vi "NI9234_SUB-VI_UserEvent.vi"(6 "Method_UsE":T3, 8 "error in (no error)":errorcluster, 11 "Cluster_UserEvent":T1) -> (0 "error out":errorcluster, 3 "user event out":refnum<user-event>)   [LabVIEW 2020]
uses:
  TYPEDEF/NI9234_TD_MethodSendEventEvent.ctl
  TYPEDEF/NI9234_TD_ClusterGUIEvents.ctl
  TYPEDEF/NI9234_TD_MethodEvent.ctl
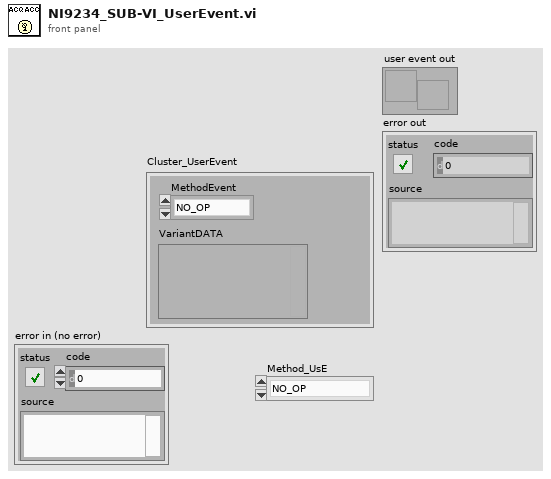
[diagram p1: front panel]
types:
  T1 = typedef "NI9234_TD_ClusterGUIEvents.ctl" = cluster{"MethodEvent":T2, "VariantDATA":variant}
  T2 = typedef "NI9234_TD_MethodEvent.ctl" = enum16{"NO_OP", "EVENTO", "ZERO_POS_REL", "ENABLE_CICLI", "CICLI_ESTENSIONE", "CICLI_RETROAZIONE", "CICLI_Numero", "CICLI_GoToMin", "CICLI_ABORT"}
  T3 = typedef "NI9234_TD_MethodSendEventEvent.ctl" = enum16{"NO_OP", "INIT", "SEND", "CLOSE"}
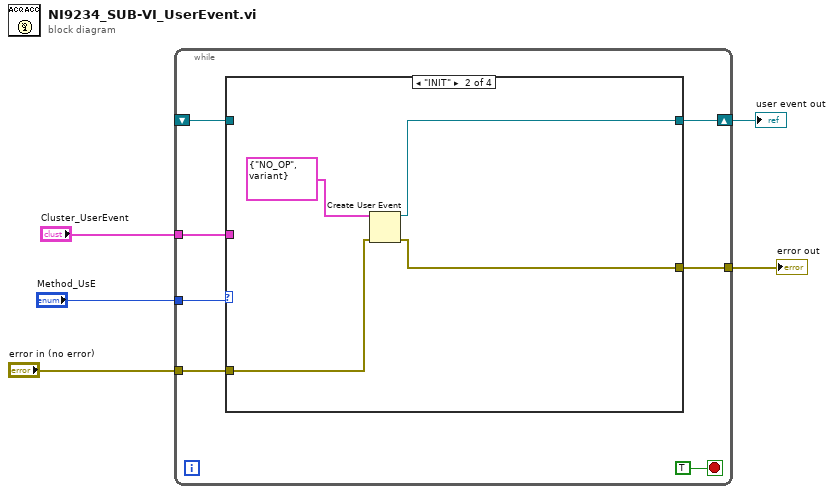
[diagram p0: block diagram]
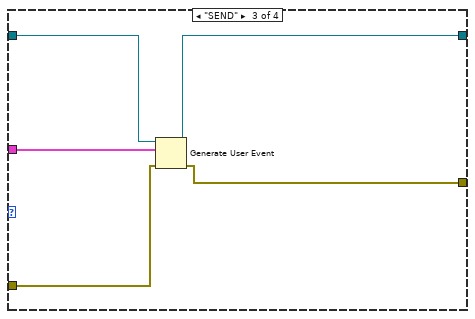
[diagram p3: hidden frame]
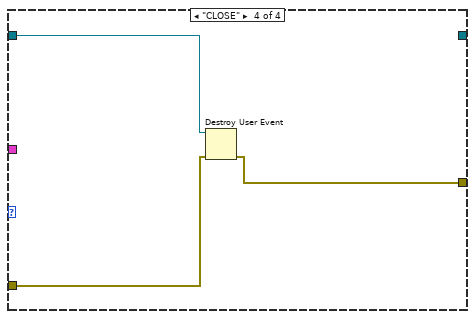
[diagram p4: hidden frame]
diagram:
  n1 = while {
    tunnel: "Method_UsE" -> [w11]
    tunnel: "Cluster_UserEvent" -> [w10]
    shift-right: [w9] -> w3
    shift-left: _ -> [w8]
    tunnel: [w7] -> w2
    tunnel: "error in (no error)" -> [w6]
    stop <- TRUE stop-if-true
    n2 = case shown="\"INIT\"" w11 {
      tunnel: w10 -> [_ _ w21 _]
      tunnel: [w14 w17 w22 _] -> w9
      tunnel: w8 -> [w14 _ w23 w26]
      tunnel: [w13 w16 w19 w25] -> w7
      tunnel: w6 -> [w13 w15 w20 w24]
      frame "NO_OP", Default {
      }
      frame "INIT" {
        n3 = Create User Event(user event datatype=T1 {"MethodEvent"=enum."NO_OP", "VariantDATA"=variant} ("Cluster_UserEvent"), error in=w15) -> (user event=w17:refnum<user-event>, error out=w16:errorcluster)
      }
      frame "SEND" {
        n4 = Generate User Event(user event=w23, event data cluster=w21, error in=w20) -> (user event out=w22:refnum<user-event>, error out=w19:errorcluster)  [unwired: 1 in]
      }
      frame "CLOSE" {
        n5 = Destroy User Event(user event=w26, error in=w24) -> (error out=w25:errorcluster)
      }
    }
  }
  "user event out" <- w3
  "error out" <- w2
